vi "Make Normal.vi"(8 "error in (no error)":errorcluster, 11 "Setup File in":refnum<class "Setup File.lvclass">) -> (0 "error out":errorcluster, 3 "Setup File out":refnum<class "Setup File.lvclass">)   [LabVIEW 2018, in "Setup File.lvclass"]
doc: "Este VI cria um arquivo texto com a configuração de normal acquisitons: VShift Speed de 0.6 us e Readout Rate de 100 KHz a 16 bit."
uses:
  Setup File.lvclass
  Setup File.lvclass/Setup File.ctl
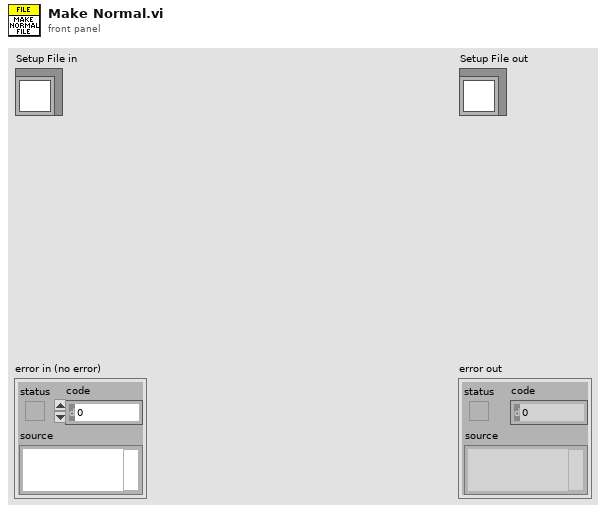
[diagram p1: front panel]
types:
  T1 = enum16{"open", "replace", "create", "open or create", "replace or create", "replace or create with confirmation"}
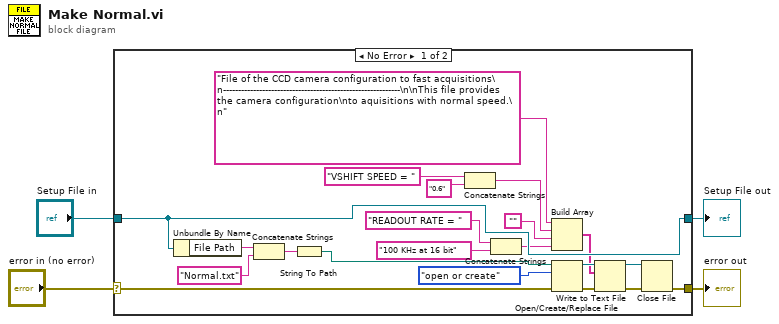
[diagram p0: block diagram]
diagram:
  n1 = case shown="No Error" "error in (no error)" {
    selector: "error in (no error)" -> [w25 w27]
    tunnel: [w22 w27] -> w3
    tunnel: [w19 w26] -> w2
    tunnel: "Setup File in" -> [w19 w26]
    frame No Error {
      n2 = Unbundle By Name(w19) -> ("File Path"=w18:string)
      n3 = Concatenate Strings(w18, "Normal.txt") -> (w17:string)
      n4 = String To Path(string=w17) -> (path=w16:path)
      n5 = Concatenate Strings("VSHIFT SPEED = ", "0.6") -> (w11:string)
      n6 = Concatenate Strings("READOUT RATE = ", "100 KHz at 16 bit") -> (w10:string)
      n7 = Build Array("File of the CCD camera configuration to fast acquisitions\n-----------------------------------------------------------\n\nThis file provides the camera configuration\nto aquisitions with normal speed.\n" ("string"), w11, "", w10) -> (w8:string[])
      n8 = Open/Create/Replace File(file path (use dialog)=w16, error in=w25, operation (0:open)=T1."open or create") -> (refnum out=w21:refnum<file>, error out=w24:errorcluster)  [unwired: 3 in, 1 out]
      n9 = Write to Text File(file (use dialog)=w21, text=w8, error in=w24) -> (refnum out=w20:refnum<file>, error out=w23:errorcluster)  [unwired: 1 in, 1 out]
      n10 = Close File(refnum=w20, error in=w23) -> (error out=w22:errorcluster)  [unwired: 1 out]
    }
    frame Error {
    }
  }
  "error out" <- w3
  "Setup File out" <- w2
